vi "Red Pitaya Test.vi"(8 "Error In":errorcluster, 10 "Server port":u16=1002, 11 "Server address":string="192.168.1.100") -> (0 "Error Out":errorcluster)   [LabVIEW 2016]
uses:
  RP Command.ctl
  RP EEPROM Calibration.ctl
  RP Write Command TCP.vi
panel:
  out "RP EEPROM Calibration":T1 {"magic" format="%x"}
  in  "New connection":bool
  out "data out":string
  in  "Command payload":u64 format="%x"
  in  "Send Button":bool
  in  "Process Stop Button":bool
  in  "Command number":T2
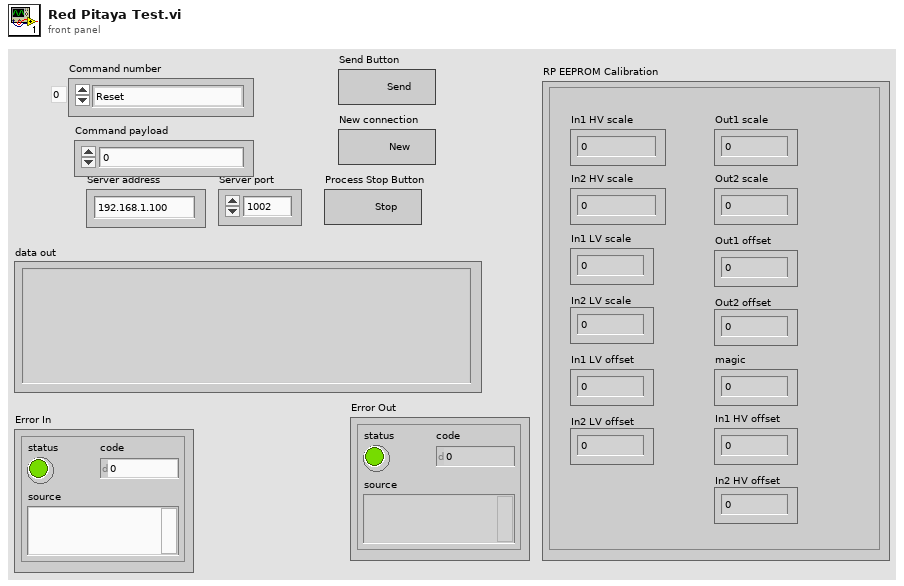
[diagram p1: front panel]
types:
  T1 = typedef "RP EEPROM Calibration.ctl" = cluster{"In1 HV scale":u32, "In2 HV scale":u32, "In1 LV scale":u32, "In2 LV scale":u32, "In1 LV offset":i32, "In2 LV offset":i32, "Out1 scale":u32, "Out2 scale":u32, "Out1 offset":i32, "Out2 offset":i32, "magic":u32, "In1 HV offset":i32, "In2 HV offset":i32}
  T2 = typedef "RP Command.ctl" = enum16{"Reset", "Read IDN", "Stop server", "Get status", "Get temperature", "Connect client", "Arm", "Software trigger", "Get whole buffer", "Get chunk", "System call", "Get config", "Set config", "Recieve data", "Recieve Calibartion", "Transmit data"}
  T3 = enum16{"big-endian, network order", "native, host order", "little-endian"}
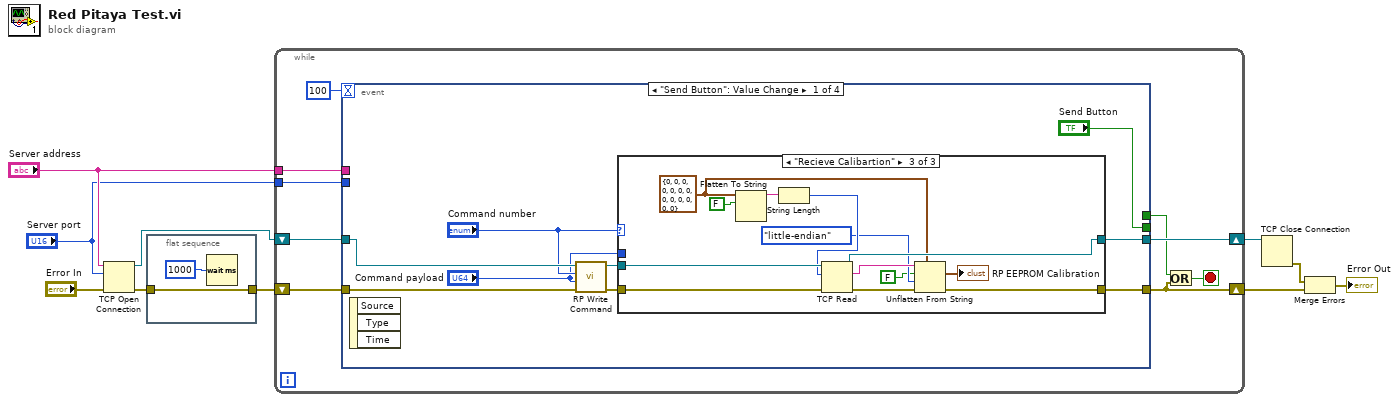
[diagram p0: block diagram]
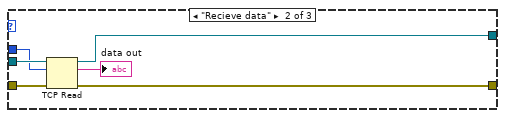
[diagram p3: hidden frame]
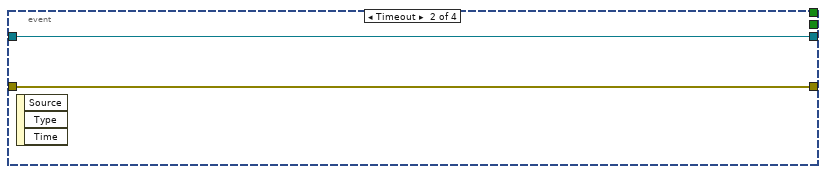
[diagram p4: hidden frame]
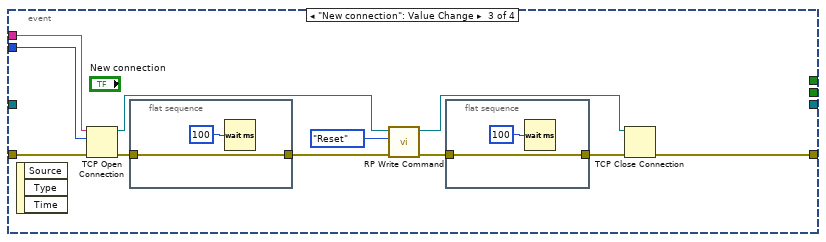
[diagram p5: hidden frame]
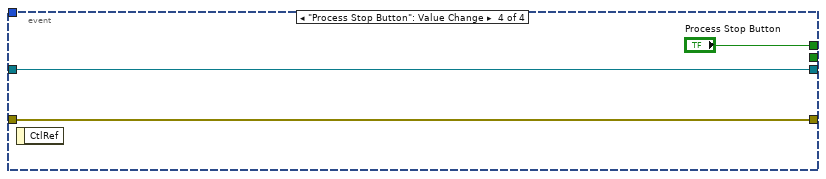
[diagram p6: hidden frame]
diagram:
  n1 = TCP Open Connection(address="Server address", remote port or service name="Server port", error in (no error)="Error In") -> (connection ID=w6:refnum<k5>, error out=w5:errorcluster)  [unwired: 2 in]
  n2 = flat-sequence {
    tunnel: w5 -> [w11]
    tunnel: [w11] -> w4
    frame #0 {
      n3 = Wait (ms)(milliseconds to wait=u32 1000) -> ()  [unwired: 1 out]
    }
  }
  n4 = while {
    shift-right: [w21] -> w8
    shift-left: w6 -> [w20]
    shift-right: [w16] -> w7
    shift-left: w4 -> [w19]
    tunnel: "Server address" -> [w14]
    tunnel: "Server port" -> [w13]
    stop <- w17 stop-if-true
    n5 = event shown="[0] \"Send Button\": Value Change" {
      selector: _ -> [_ _ _ _]
      dyn-events: _ -> [_ _ _ _]
      timeout: 100 -> [_ _ _ _]
      tunnel: [w23 w53 _ w69] -> w21
      tunnel: [w22 w52 w54 w70] -> w16
      tunnel: w20 -> [w30 w53 _ w69]
      tunnel: w19 -> [w29 w52 w64 w70]
      tunnel: [_ _ _ "Process Stop Button"] -> w18
      tunnel: ["Send Button" _ _ _] -> _
      tunnel: w14 -> [_ _ w63 _]
      tunnel: w13 -> [_ _ w62 _]
      event "Send Button": Value Change {
        n6 = event-data() -> ()  [unwired: 1 in, 3 out]
        n7 = call-poly "RP Write Command.vi"("Error In"=w29, "Command payload"="Command payload", "Command number"="Command number", "connection ID"=w30) -> ("Error Out"=w27:errorcluster, "connection ID out"=w24:refnum<k5>)  [unwired: 5 in, 1 out]
        n8 = case shown="\"Recieve Calibartion\"" "Command number" {
          tunnel: w27 -> [w31 w38 w51]
          tunnel: "Command payload" -> [_ w36 _]
          tunnel: w24 -> [w32 w37 w50]
          tunnel: [w32 w35 w49] -> w23
          tunnel: [w31 w34 w41] -> w22
          frame "Reset", Default {
          }
          frame "Recieve data" {
            n9 = TCP Read(connection ID=w37, bytes to read=w36, error in (no error)=w38) -> (connection ID out=w35:refnum<k5>, data out=→"data out":string, error out=w34:errorcluster)  [unwired: 2 in]
          }
          frame "Recieve Calibartion" {
            w44 = T1 {"In1 HV scale"=0, "In2 HV scale"=0, "In1 LV scale"=0, "In2 LV scale"=0, "In1 LV offset"=0, "In2 LV offset"=0, "Out1 scale"=0, "Out2 scale"=0, "Out1 offset"=0, "Out2 offset"=0, "magic"=0, "In1 HV offset"=0, "In2 HV offset"=0} ("RP EEPROM Calibration")
            n10 = Flatten To String(anything=w44, prepend array or string size? (T)=FALSE) -> (data string=w47:string)  [unwired: 2 in, 2 out]
            n11 = String Length(string=w47) -> (length=w46:i32)
            n12 = TCP Read(connection ID=w50, bytes to read=w46, error in (no error)=w51) -> (connection ID out=w49:refnum<k5>, data out=w45:string, error out=w42:errorcluster)  [unwired: 2 in]
            n13 = Unflatten From String(type=w44, binary string=w45, data includes array or string size? (T)=FALSE, byte order (0:big-endian, network order)=T3."little-endian", error in (no error)=w42) -> (value=→"RP EEPROM Calibration":T1, error out=w41:errorcluster)  [unwired: 1 out]
          }
        }
      }
      event Timeout {
        n14 = event-data() -> ()  [unwired: 1 in, 3 out]
      }
      event "New connection": Value Change {
        n15 = event-data() -> ()  [unwired: 1 in, 3 out]
        n16 = TCP Open Connection(address=w63, remote port or service name=w62, error in (no error)=w64) -> (connection ID=w59:refnum<k5>, error out=w61:errorcluster)  [unwired: 2 in]
        n17 = flat-sequence {
          tunnel: w61 -> [w67]
          tunnel: [w67] -> w60
          frame #0 {
            n18 = Wait (ms)(milliseconds to wait=u32 100) -> ()  [unwired: 1 out]
          }
        }
        n19 = call-poly "RP Write Command.vi"("Error In"=w60, "Command number"=RP_Command."Reset", "connection ID"=w59) -> ("Error Out"=w57:errorcluster, "connection ID out"=w55:refnum<k5>)  [unwired: 6 in, 1 out]
        n20 = flat-sequence {
          tunnel: w57 -> [w65]
          tunnel: [w65] -> w56
          frame #0 {
            n21 = Wait (ms)(milliseconds to wait=u32 100) -> ()  [unwired: 1 out]
          }
        }
        n22 = TCP Close Connection(connection ID=w55, error in (no error)=w56) -> (error out=w54:errorcluster)  [unwired: 1 in, 1 out]
      }
      event "Process Stop Button": Value Change {
        n23 = event-data() -> ()  [unwired: 1 in, 1 out]
      }
    }
    n24 = Or(x=w18, y=w16) -> (x .or. y?=w17:bool)
  }
  n25 = TCP Close Connection(connection ID=w8) -> (error out=w10:errorcluster)  [unwired: 2 in, 1 out]
  n26 = Merge Errors(w10, w7) -> (→"Error Out":errorcluster)
